vi "mhk_velmex.vi"() -> ()   [LabVIEW 2010]
panel:
  in  "VISA resource name":refnum<visa-resource-name>
  out "Command String":string
  in  "Number of Steps":u32(knob)=1 min=1 max=100000 step=1 scale=1.0..100000.0
  in  "Direction":bool
  in  "Motor Speed\n(Steps/sec)":i32(knob)=2000 min=2000 max=8000 scale=2000.0..8000.0
  in  "Motor Number":dbl=1.0 min=1.0 max=4.0 step=1.0
  # "Negative"
  # "Positive"
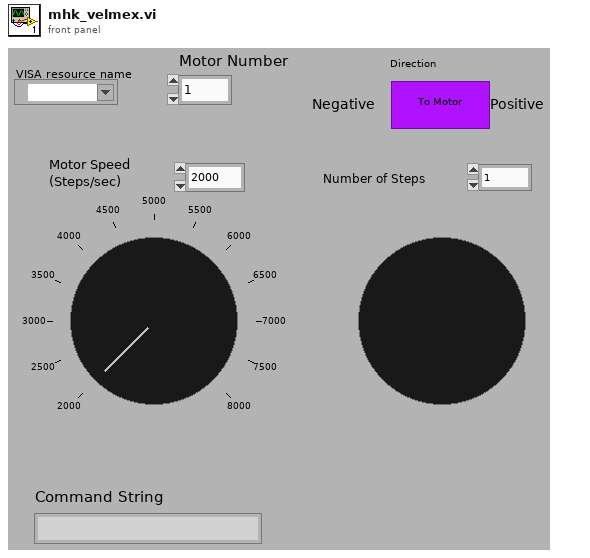
[diagram p1: front panel]
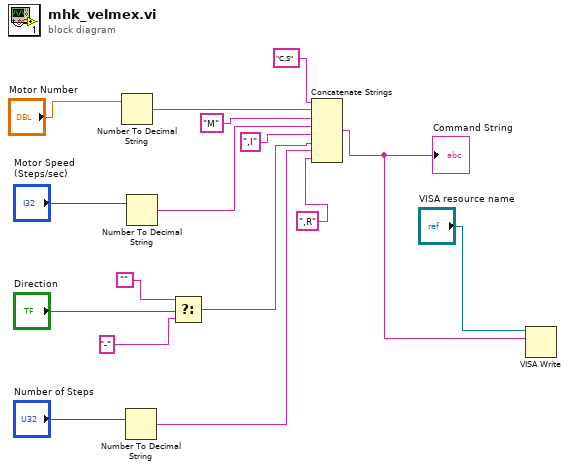
[diagram p0: block diagram]
diagram:
  n1 = Number To Decimal String(number="Motor Number") -> (decimal integer string=w9:string)  [unwired: 1 in]
  n2 = Number To Decimal String(number="Number of Steps") -> (decimal integer string=w4:string)  [unwired: 1 in]
  n3 = Number To Decimal String(number="Motor Speed\n(Steps/sec)") -> (decimal integer string=w7:string)  [unwired: 1 in]
  n4 = Select(t="", s="Direction", f="-") -> (s? t:f=w5:string)
  n5 = Concatenate Strings("C,S", w9, "M", w7, ",I", w5, w4, ",R") -> (w2:string)
  "Command String" <- w2
  n6 = VISA Write(VISA resource name="VISA resource name", write buffer=w2) -> ()  [unwired: 1 in, 3 out]
